vi "Set System Channels Group Properties.vi"(8 "error in (no error)":errorcluster, 10 "Logger Parameters":T1, 11 "Refnum in":refnum<k34>) -> (0 "error out":errorcluster, 3 "Refnum out":refnum<k34>)   [LabVIEW 2020, in "Telemetry Engine.lvlib"]
uses:
  Telemetry Engine.lvlib
  Types/Logger Data.ctl
  Types/Async Logger State Data.ctl
  Types/System Channels.ctl
  Types/Target Info.ctl
  Shared/Constants.vi
  Shared/Telemetry Shared.lvlib
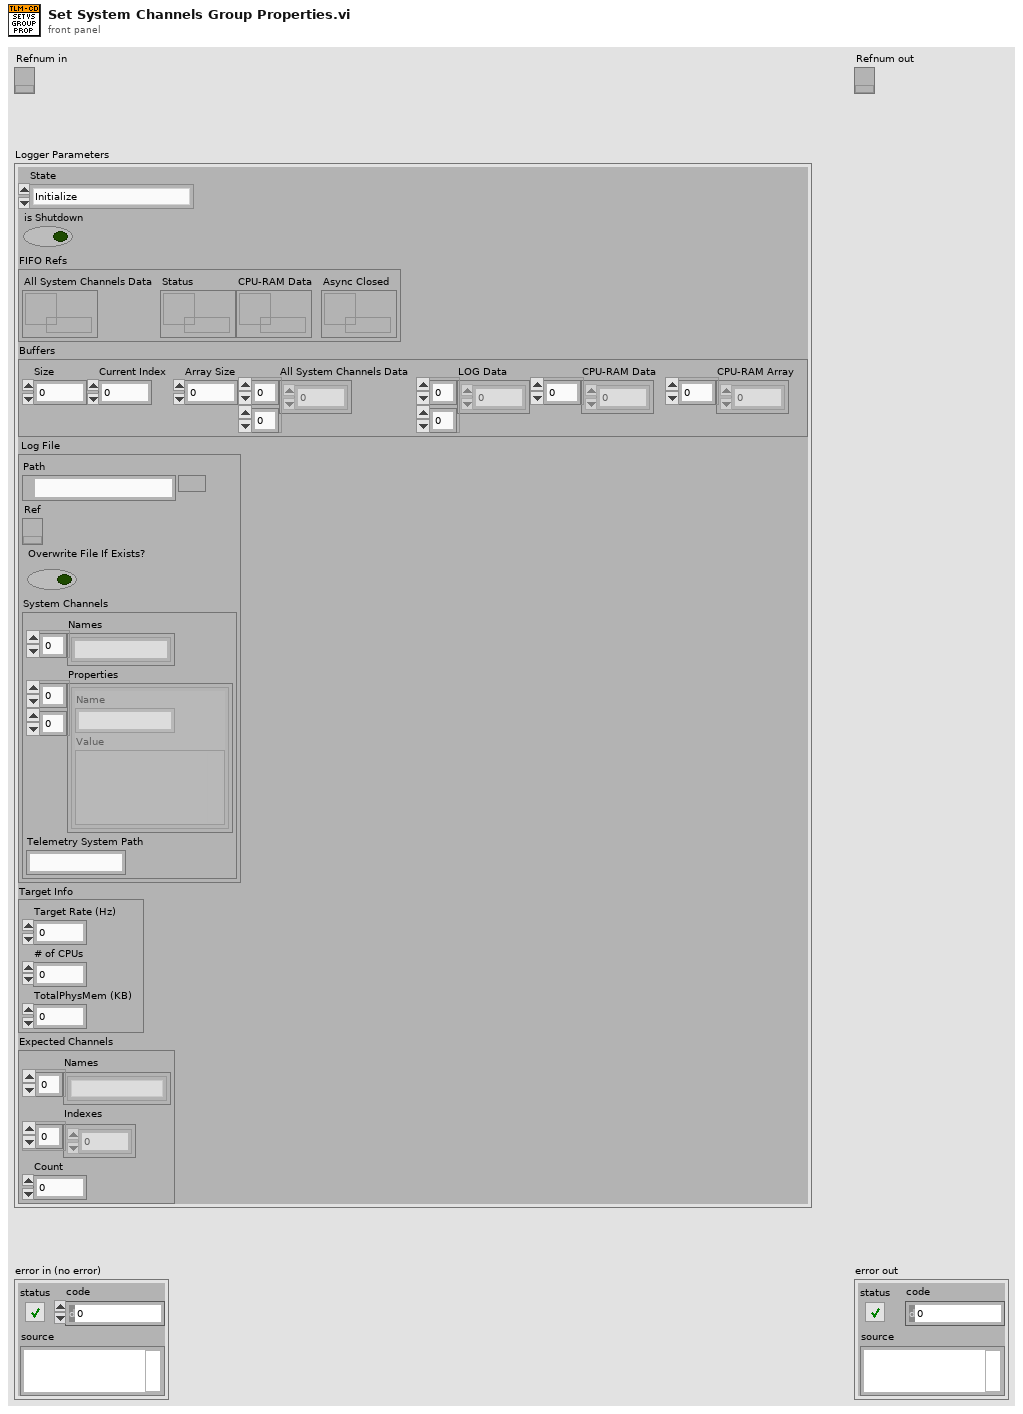
[diagram p1: front panel]
types:
  T1 = typedef "Telemetry Engine.lvlib/Logger Data.ctl" = cluster{"State":T2, "is Shutdown":bool, "FIFO Refs":cluster{"All System Channels Data":refnum<k33>, "Status":refnum<k33>, "CPU-RAM Data":refnum<k33>, "Async Closed":refnum<k33>}, "Buffers":cluster{"Size":i32, "Current Index":i32, "Array Size":i32, "All System Channels Data":dbl[][], "LOG Data":dbl[][], "CPU-RAM Data":dbl[], "CPU-RAM Array":dbl[]}, "Log File":cluster{"Path":path, "Ref":refnum<k34>, "Overwrite File If Exists?":bool, "System Channels":T3}, "Target Info":T4, "Expected Channels":cluster{"Names":string[], "Indexes":i32[], "Count":i32}}
  T2 = typedef "Telemetry Engine.lvlib/Async Logger State Data.ctl" = enum16{"Initialize", "Read System Channels FIFO", "Filter System Channels", "Read CPU-RAM FIFO", "Log Data", "Shutdown"}
  T3 = typedef "Telemetry Engine.lvlib/System Channels.ctl" = cluster{"Names":string[], "Properties":cluster{"Name":string, "Value":variant}[][], "Telemetry System Path":string}
  T4 = typedef "Telemetry Engine.lvlib/Target Info.ctl" = cluster{"Target Rate (Hz)":dbl, "# of CPUs":u32, "TotalPhysMem (KB)":dbl}
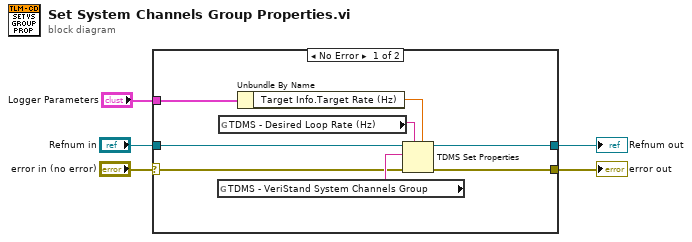
[diagram p0: block diagram]
diagram:
  n1 = case shown="No Error" "error in (no error)" {
    selector: "error in (no error)" -> [w11 w15]
    tunnel: "Logger Parameters" -> [w7 _]
    tunnel: "Refnum in" -> [w13 w14]
    tunnel: [w9 w14] -> w4
    tunnel: [w8 w15] -> w3
    frame No Error {
      n2 = global read "Constants.vi" "TDMS - VeriStand System Channels Group"() -> (w12:string)
      n3 = global read "Constants.vi" "TDMS - Desired Loop Rate (Hz)"() -> (w10:string)
      n4 = Unbundle By Name(w7) -> ("Target Info.Target Rate (Hz)"=w6:dbl)
      n5 = TDMS Set Properties(5:w6, 7:w10, 8:w11, 10:w12, 11:w13) -> (0:w8:errorcluster, 3:w9:refnum<k34>)  [unwired: 1 in, 2 out]
    }
    frame Error {
    }
  }
  "Refnum out" <- w4
  "error out" <- w3
